vi "SubdevideInt.vi"(2 "Input String":string, 3 "Delimiter":string=" ", 4 "INT or String":string=" ") -> (0 "Output Array":string[](array[string]), 1 "Output Array":i32[](array[numeric]))   [LabVIEW 2011]
doc: "This VI subdevide a string to an array with space as a delimiter."
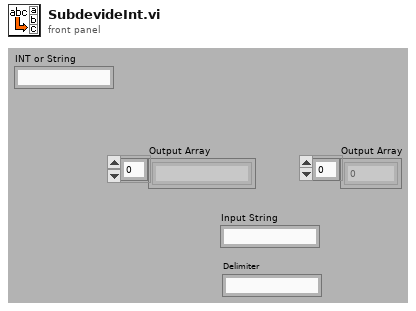
[diagram p1: front panel]
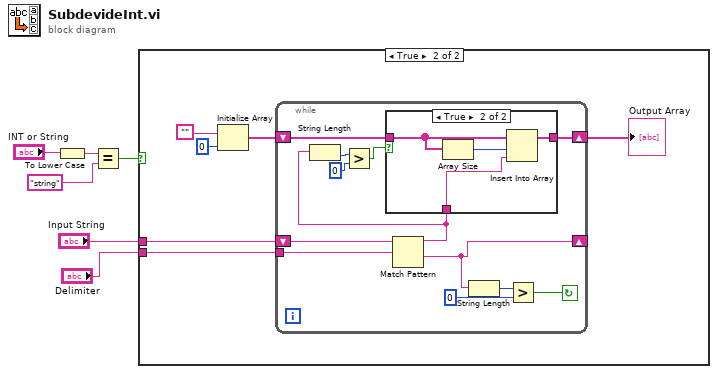
[diagram p0: block diagram]
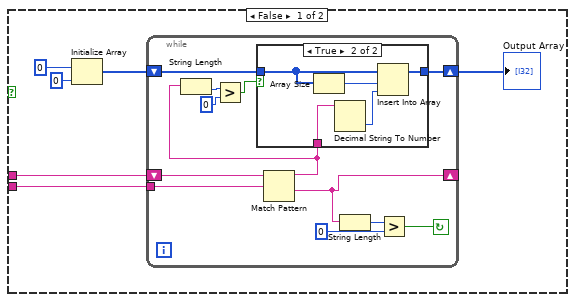
[diagram p2: hidden frame]
diagram:
  n1 = To Lower Case(string="INT or String") -> (all lower case string=w3:string)
  n2 = Equal?(x=w3, y="string") -> (x = y?=w1:bool)
  n3 = case shown="True" w1 {
    tunnel: "Input String" -> [w10 w32]
    tunnel: "Delimiter" -> [w7 w31]
    frame False {
      n4 = Initialize Array(0, 0 ("dimension size")) -> (w11:i32[])
      n5 = while {
        shift-right: [w24] -> w8
        shift-left: w11 -> [w23]
        shift-right: [w20] -> _
        shift-left: w10 -> [w22]
        tunnel: w7 -> [w13]
        stop <- w18 continue-if-true
        n6 = Match Pattern(string=w22, regular expression=w13) -> (before substring=w14:string, after substring=w20:string)  [unwired: 1 in, 2 out]
        n7 = String Length(string=w14) -> (length=w17:i32)
        n8 = Greater?(x=w17, y=0) -> (0:w16:bool)
        n9 = case shown="True" w16 {
          tunnel: [w25 w30] -> w24
          tunnel: w23 -> [w25 w29]
          tunnel: w14 -> [_ w26]
          frame False {
          }
          frame True {
            n10 = Array Size(array=w29) -> (size(s)=w28:i32)
            n11 = Decimal String To Number(string=w26) -> (number=w27:i32)  [unwired: 2 in, 1 out]
            n12 = Insert Into Array(array=w29, index=w28, new element=w27) -> (w30:i32[])
          }
        }
        n13 = String Length(string=w20) -> (length=w21:i32)
        n14 = Greater?(x=w21, y=0) -> (0:w18:bool)
      }
      "Output Array" <- w8
    }
    frame True {
      n15 = Initialize Array("", 0 ("dimension size")) -> (w35:string[])
      n16 = while {
        shift-right: [w48] -> w33
        shift-left: w35 -> [w47]
        shift-right: [w44] -> _
        shift-left: w32 -> [w46]
        tunnel: w31 -> [w37]
        stop <- w42 continue-if-true
        n17 = Match Pattern(string=w46, regular expression=w37) -> (before substring=w38:string, after substring=w44:string)  [unwired: 1 in, 2 out]
        n18 = String Length(string=w38) -> (length=w41:i32)
        n19 = Greater?(x=w41, y=0) -> (0:w40:bool)
        n20 = case shown="True" w40 {
          tunnel: [w49 w53] -> w48
          tunnel: w47 -> [w49 w52]
          tunnel: w38 -> [_ w50]
          frame False {
          }
          frame True {
            n21 = Array Size(array=w52) -> (size(s)=w51:i32)
            n22 = Insert Into Array(array=w52, index=w51, new element=w50) -> (w53:string[])
          }
        }
        n23 = String Length(string=w44) -> (length=w45:i32)
        n24 = Greater?(x=w45, y=0) -> (0:w42:bool)
      }
      "Output Array" <- w33
    }
  }
